vi "Write Enable.vi"(8 "error in (no error)":errorcluster, 10 "Enable":refnum<k21>, 11 "cCRDS_new in":refnum<class "cCRDS.lvclass">=refnum) -> (0 "error out":errorcluster, 3 "cCRDS_new out":refnum<class "cCRDS.lvclass">)   [LabVIEW 2015, in "cCRDS.lvclass"]
uses:
  cCRDS.lvclass
  cCRDS.lvclass/cCRDS.ctl
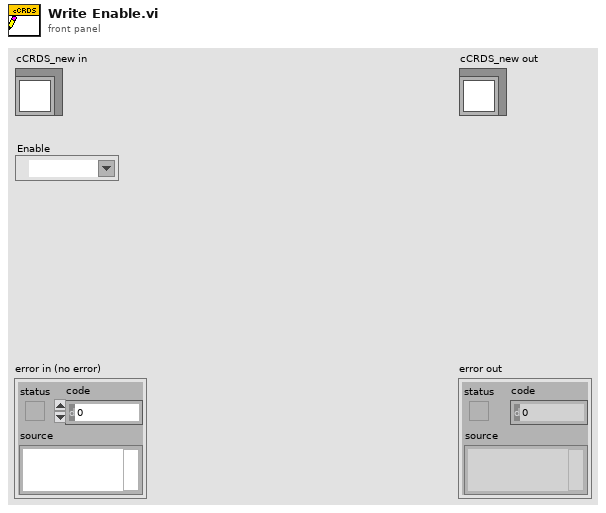
[diagram p1: front panel]
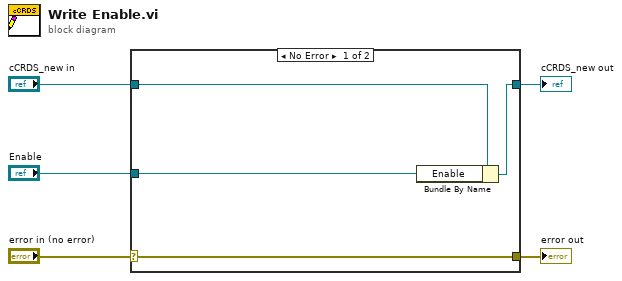
[diagram p0: block diagram]
diagram:
  n1 = case shown="No Error" "error in (no error)" {
    selector: "error in (no error)" -> [w9 w10]
    tunnel: [w9 w10] -> w4
    tunnel: [w7 w11] -> w2
    tunnel: "cCRDS_new in" -> [w8 w11]
    tunnel: "Enable" -> [w6 _]
    frame No Error {
      n2 = Bundle By Name(cluster=w8, "Enable"=w6) -> (w7:refnum<class "cCRDS.lvclass">)
    }
    frame Error {
    }
  }
  "error out" <- w4
  "cCRDS_new out" <- w2
